vi "ReadI64.vi"(8 "error in (no error)":errorcluster, 10 "Start address":string, 11 "MelsecTCP in":refnum<class "Abs Controler.lvclass">) -> (0 "error out":errorcluster, 2 "Data":i64, 3 "MelsecTCP out":refnum<class "Abs Controler.lvclass">)   [LabVIEW 2020, in "HslCommunication.lvlib" / "Abs Controler.lvclass"]
uses:
  Abs Controler.lvclass
  E:/Git/Libraries/develop/HslCommunication/_Dependenciecs/HslCommunication.dll
  _Dependenciecs/HslCommunication.dll
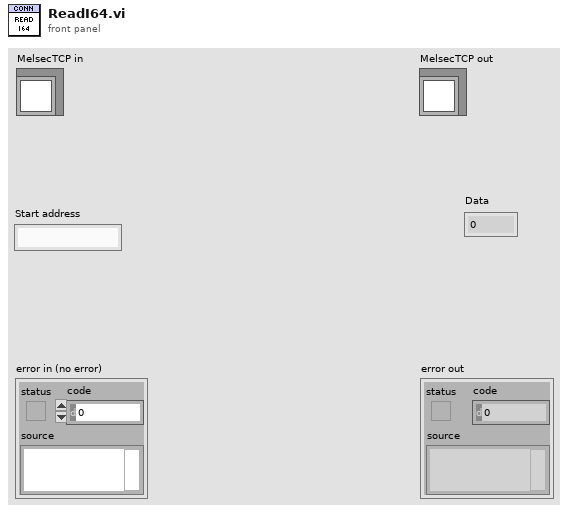
[diagram p1: front panel]
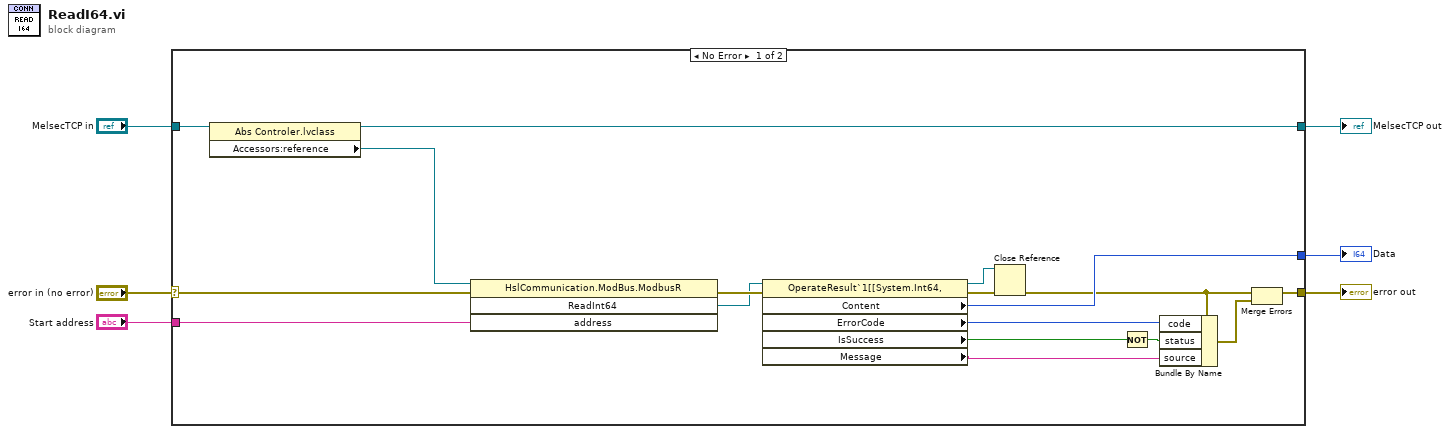
[diagram p0: block diagram]
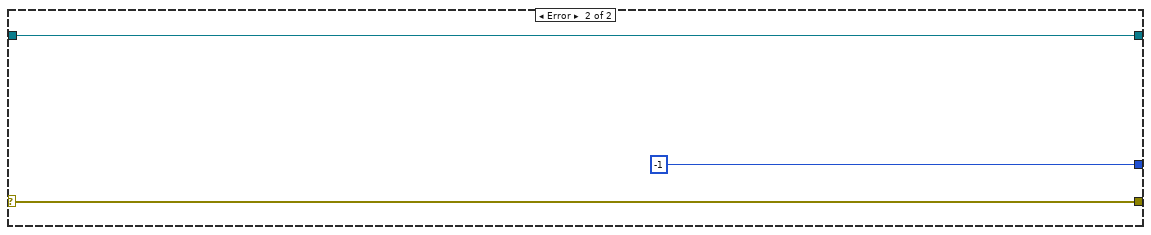
[diagram p2: hidden frame]
diagram:
  n1 = case shown="No Error" "error in (no error)" {
    selector: "error in (no error)" -> [w7 w26]
    tunnel: "MelsecTCP in" -> [w23 w25]
    tunnel: [w15 w25] -> w2
    tunnel: "Start address" -> [w14 _]
    tunnel: [w21 w26] -> w3
    tunnel: [w22 -1 ("Content")] -> w1
    frame No Error {
      n2 = property class="Abs Controler.lvclass"(reference=w23) -> (reference out=w15:refnum<class "Abs Controler.lvclass">, "Accessors:reference"=w8:refnum<k24>)  [unwired: 1 in, 1 out]
      n3 = invoke class="HslCommunication.ModBus.ModbusR" method="ReadInt64"(reference=w8, error in=w7, "address"=w14) -> (error out=w12:errorcluster, "ReadInt64"=w10:refnum<k24>)  [unwired: 1 in, 2 out]
      n4 = property class="OperateResult`1[[System.Int64, "(reference=w10, error in=w12) -> (reference out=w9:refnum<k24>, error out=w11:errorcluster, "Content"=w22:i64, "ErrorCode"=w20:i32, "IsSuccess"=w19:bool, "Message"=w18:string)
      n5 = Close Reference(reference=w9, error in (no error)=w11) -> (error out=w17:errorcluster)
      n6 = Not(x=w19) -> (.not. x?=w13:bool)
      n7 = Bundle By Name(cluster=w17, "code"=w20, "status"=w13, "source"=w18) -> (w16:errorcluster)
      n8 = Merge Errors(w17, w16) -> (w21:errorcluster)
    }
    frame Error {
    }
  }
  "error out" <- w3
  "MelsecTCP out" <- w2
  "Data" <- w1
